vi "Parse From String.vi"(8 "error in (no error)":errorcluster, 9 "Request String":string) -> (0 "error out":errorcluster, 3 "Request out":refnum<class "Request.lvclass">)   [LabVIEW 2020, in "HTTP Utils.lvlib" / "Request.lvclass"]
uses:
  Request.lvclass
  <vilib>/IlluminatedG/lv-stream/stream/StringStream/StringStream.lvclass
  C:/Program Files (x86)/National Instruments/LabVIEW 2020/vi.lib/IlluminatedG/lv-stream/stream/Stream.lvclass
  Request.lvclass/Request.ctl
  C:/Program Files (x86)/National Instruments/LabVIEW 2020/vi.lib/IlluminatedG/lv-stream/stream/StringStream/StringStream.lvclass
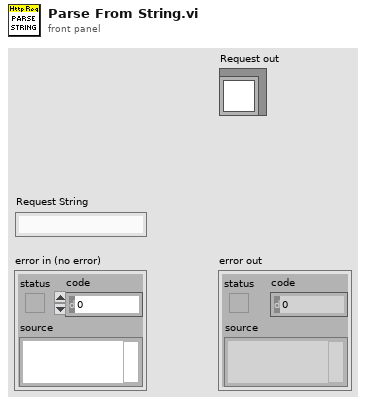
[diagram p1: front panel]
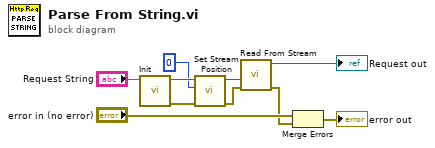
[diagram p0: block diagram]
diagram:
  n1 = call <vilib>:"Init.vi"("Initial String (Empty)"="Request String") -> ("error out"=w3:errorcluster, "StringStream out"=w5:refnum<class "StringStream.lvclass">)  [unwired: 9 in]
  n2 = call-dynamic "Set Stream Position.vi"("error in (no error)"=w3, "Read Position"=i64 0, "StringStream in"=w5) -> ("error out"=w1:errorcluster, "StringStream out"=w2:refnum<class "StringStream.lvclass">)  [unwired: 7 in]
  n3 = call "Read From Stream.vi"("error in (no error)"=w1, "Stream in"=w2) -> ("error out"=w6:errorcluster, "Request out"=→"Request out":refnum<class "Request.lvclass">)  [unwired: 7 in, 1 out]
  n4 = Merge Errors("error in (no error)", w6) -> (→"error out":errorcluster)
